vi "Abort.vi"(8 "error in (no error)":errorcluster, 11 "NI SMU in":refnum<class "NI SMU.lvclass">) -> (0 "error out":errorcluster, 3 "NI SMU out":refnum<class "NI SMU.lvclass">)   [LabVIEW 2020, in "NI SMU.lvlib" / "NI SMU.lvclass"]
uses:
  NI SMU.lvclass
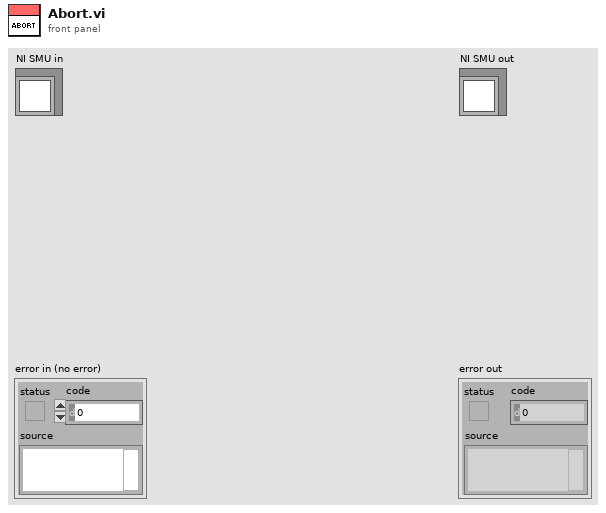
[diagram p1: front panel]
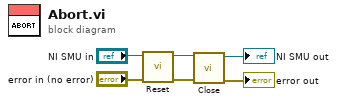
[diagram p0: block diagram]
diagram:
  n1 = call-dynamic "Reset.vi"("error in (no error)"="error in (no error)", "NI SMU in"="NI SMU in") -> ("error out"=w4:errorcluster, "NI SMU out"=w3:refnum<class "NI SMU.lvclass">)  [unwired: 8 in]
  n2 = call-dynamic "Close.vi"("error in (no error)"=w4, "NI SMU in"=w3) -> ("error out"=→"error out":errorcluster, "NI SMU out"=→"NI SMU out":refnum<class "NI SMU.lvclass">)  [unwired: 8 in]
